vi "0 - JudgeLogValueChange.vi"(8 "error in (no error)":errorcluster, 11 "String In":string) -> (0 "error out":errorcluster, 2 "Value Changed?":bool, 3 "String Out":string)   [LabVIEW 2017]
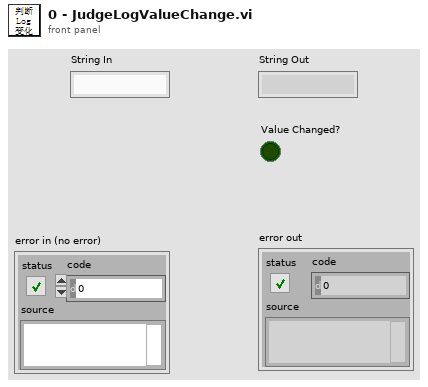
[diagram p1: front panel]
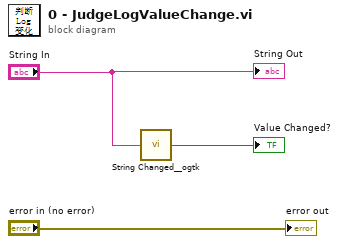
[diagram p0: block diagram]
diagram:
  n1 = call "String Changed__ogtk.vi"("String"="String In") -> ("Changed"=→"Value Changed?":bool)
  "String Out" <- "String In"
  "error out" <- "error in (no error)"
